vi "Configure Power Ramp Mode.vi"(8 "error in (no error)":errorcluster, 10 "power ramp mode":u8(ring) items=["off", "ramp up", "ramp up and down", "ramp down"], 11 "HFP Gen in":refnum<class "PL HFP Generator.lvclass">) -> (0 "error out":errorcluster, 3 "HFP Gen out":refnum<class "PL HFP Generator.lvclass">)   [LabVIEW 2015, in "PL HFP Generator.lvclass"]
doc: "Configures power ramp mode."
uses:
  PL HFP Generator.lvclass
  <vilib>/plasmapper/PL Modbus Client/PL Modbus Client.lvclass
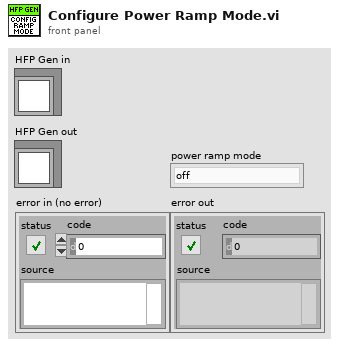
[diagram p1: front panel]
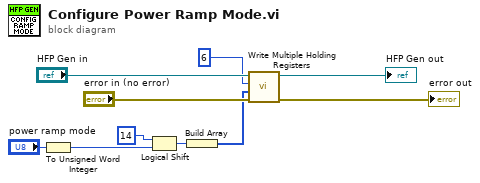
[diagram p0: block diagram]
diagram:
  n1 = To Unsigned Word Integer(number="power ramp mode") -> (unsigned 16bit integer=w3:u16)
  n2 = Logical Shift(y=i16 14, x=w3) -> (x << y=w2:u16)
  n3 = Build Array(w2) -> (w5:u16[])
  n4 = call <vilib>:"Write Multiple Holding Registers.vi"("error in (no error)"="error in (no error)", "values"=w5, "address"=u16 6, "MODBUS in"="HFP Gen in") -> ("error out"=→"error out":errorcluster, "MODBUS out"=→"HFP Gen out":refnum<class "PL HFP Generator.lvclass">)  [unwired: 6 in]
